vi "DaNISim.vi"(4 "Sonar offset angle":dbl, 5 "Action":enum16{"Init", "Run", "Release"}(ring), 6 "Sonar angle":dbl, 7 "Mode Select":T1(ring), 8 "error in (no error)":errorcluster, 9 "IP Adress":T2, 10 "Ul":dbl, 11 "Ur":dbl) -> (0 "error out":errorcluster, 1 "Sonar distance":dbl, 2 "OmegaL":dbl, 3 "OmegaR":dbl)   [LabVIEW 2016]
uses:
  <vilib>/userdefined/High Color/nirio_resource_hc.ctl
  <vilib>/robotics/Starter Kit/2.0/Sim Host Interface/NI_Robotics_Starter Kit Host_Sim_2.0.lvclass
  C:/Program Files (x86)/National Instruments/LabVIEW 2016/vi.lib/robotics/Starter Kit/Host Interface/NI_Robotics_Starter Kit Host.lvclass
  <vilib>/FPGAPlugInAG/sbRIO-9632/niLvFpga_Open_sbRIO-9632.vi
  <vilib>/rvi/interface/common/dynamic/niFpgaDynamicAddResources.vi
  <vilib>/Utility/error.llb/Error Cluster From Error Code.vi
  <vilib>/rvi/errors/niLvFpgaAdjustHostInterfaceError.vi
  <vilib>/FPGAPlugInAG/Dynamic/niLvFpga_Close_Dynamic.vi
  <vilib>/rvi/interface/nirviOpenFPGA/nirviOpenFPGA.xnode
  FPGA Bitfiles/StarterKit2.0Cus_FPGATarget_StarterKit2.0Cus_pLn805qeh78.lvbitx
  <vilib>/rvi/interface/nirviReadWriteControl/nirviReadWriteControl.xnode
  <vilib>/rvi/interface/nirviCloseFPGA/nirviCloseFPGA.xnode
  NiFpgaLv.dll
  <vilib>/rvi/interface/Simulation/niFpgaSimulationCallBeginRW.vi
  <vilib>/robotics/Simulator/NI_Robotics_Simulator.lvlib
  <vilib>/robotics/Starter Kit/Host Interface/NI_Robotics_Starter Kit Host.lvclass
panel:
  in  "N":i32=100
  in  "J":dbl=0.03
  in  "L":dbl=0.1825
  in  "R":dbl=0.046
  in  "M":dbl=3.0
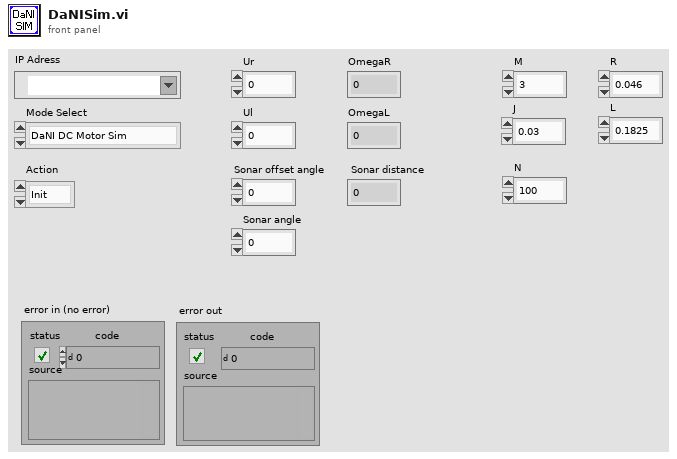
[diagram p1: front panel]
types:
  T1 = enum16{"DaNI DC Motor Sim", "DaNI Simulation", "DaNI Robot"}
  T2 = typedef "nirio_resource_hc.ctl" = tag
  T3 = cluster{"period (uSec)":u32, "pulse width (uSec)":u32}
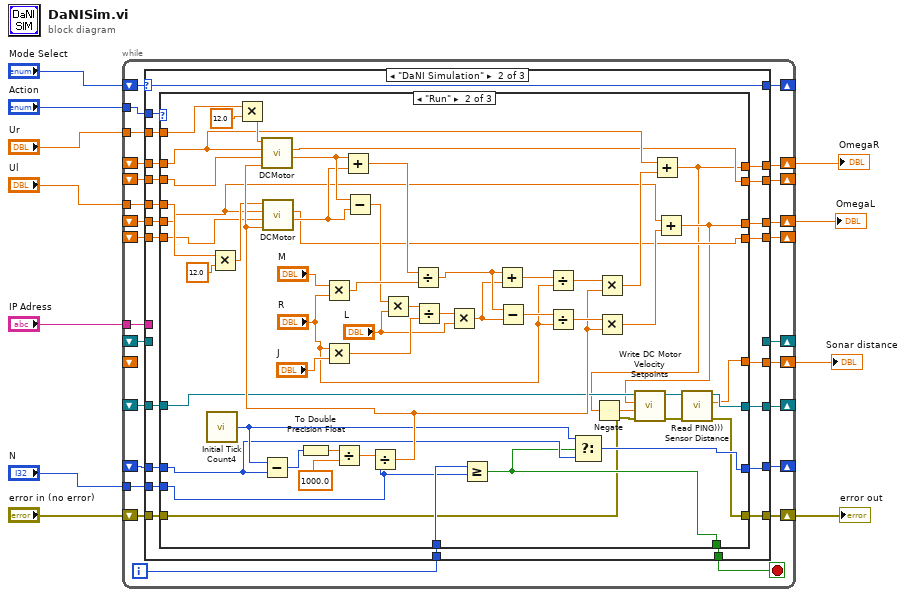
[diagram p0: block diagram]
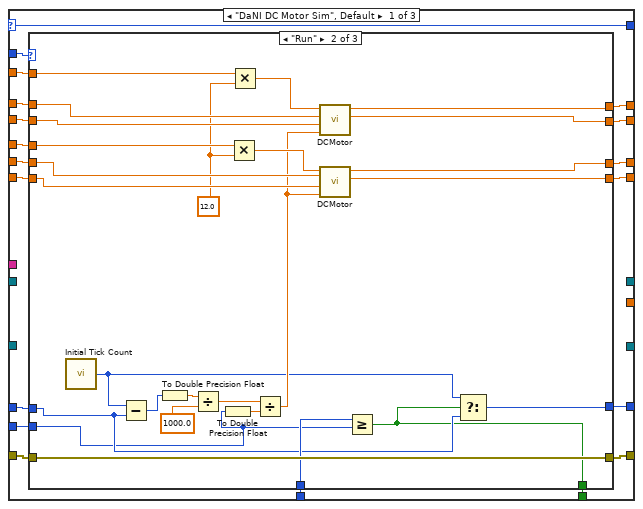
[diagram p2: hidden frame]
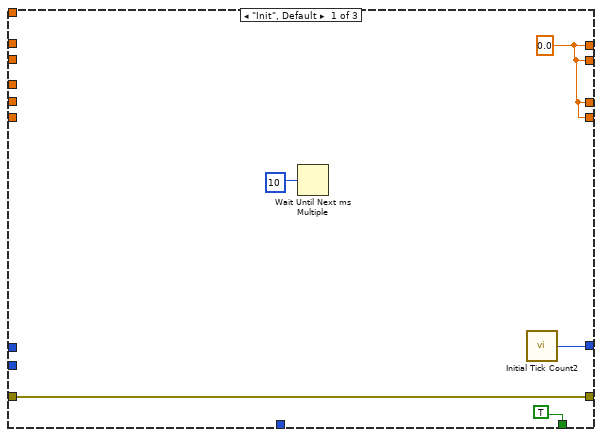
[diagram p3: hidden frame]
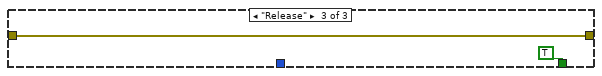
[diagram p4: hidden frame]
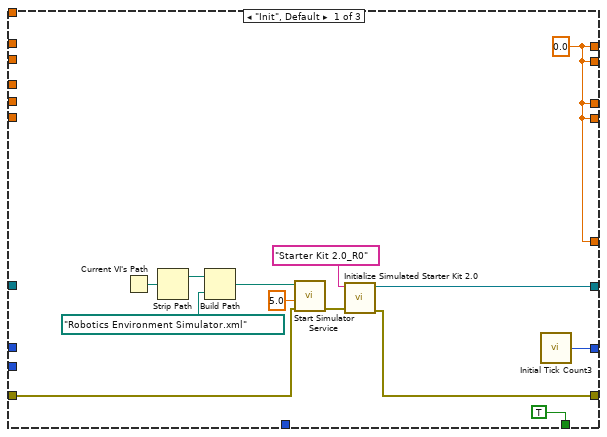
[diagram p5: hidden frame]
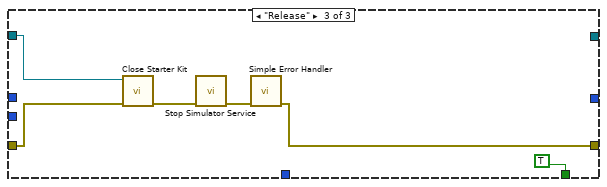
[diagram p6: hidden frame]
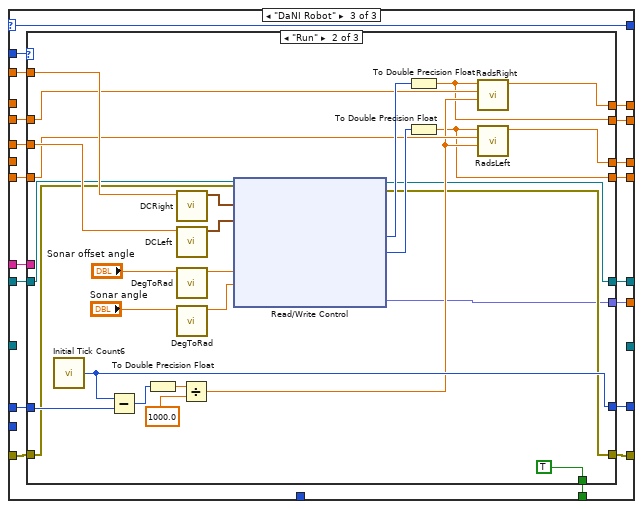
[diagram p7: hidden frame]
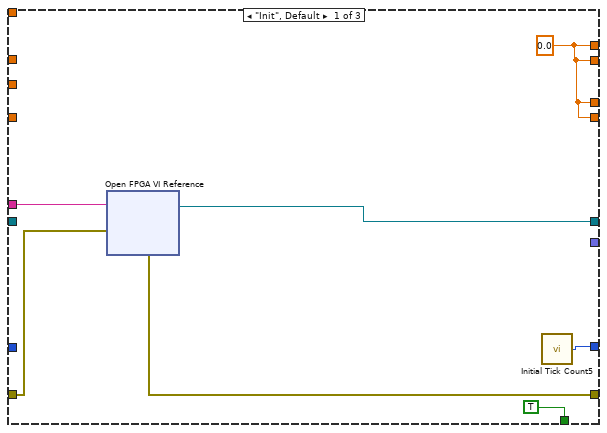
[diagram p8: hidden frame]
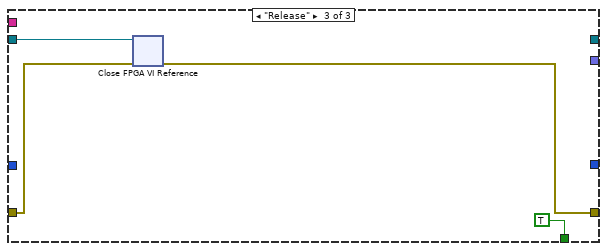
[diagram p9: hidden frame]
diagram:
  n1 = while {
    shift-right: [w35] -> w5
    shift-left: _ -> [w28]
    shift-right: [w34] -> _
    shift-left: _ -> [w27]
    tunnel: "Ur" -> [w29]
    shift-right: [w33] -> w4
    shift-left: _ -> [w25]
    shift-right: [w32] -> _
    shift-left: _ -> [w24]
    tunnel: "Ul" -> [w26]
    shift-right: [w30] -> _
    shift-left: _ -> [w31]
    shift-right: [w20] -> _
    shift-left: _ -> [w19]
    tunnel: "IP Adress" -> [w21]
    tunnel: "Action" -> [w36]
    shift-right: [w18] -> _
    shift-left: "Mode Select" -> [w37]
    tunnel: "N" -> [w17]
    shift-right: [w16] -> _
    shift-left: _ -> [w15]
    shift-right: [w14] -> w2
    shift-left: _ -> [_]
    shift-right: [w13] -> w1
    shift-left: "error in (no error)" -> [w12]
    i -> [w22]
    stop <- w23 stop-if-true
    n2 = case shown="\"DaNI Simulation\"" w37 {
      selector: w37 -> [w40 w94 w185]
      tunnel: w36 -> [w56 w107 w196]
      tunnel: [w55 w111 w202] -> w35
      tunnel: [w54 w110 w201] -> w34
      tunnel: [w53 w109 w200] -> w33
      tunnel: [w52 w108 w199] -> w32
      tunnel: w12 -> [w43 w105 w198]
      tunnel: [w42 w104 w197] -> w13
      tunnel: w31 -> [w51 w96 w188]
      tunnel: [w50 w103 w195] -> w30
      tunnel: w29 -> [w49 w102 w192]
      tunnel: w28 -> [w48 w101 _]
      tunnel: w27 -> [w47 w100 w190]
      tunnel: w26 -> [w46 w99 w191]
      tunnel: w25 -> [w45 w97 _]
      tunnel: w24 -> [w44 w98 w189]
      tunnel: [w41 w106 w186] -> w23
      tunnel: w22 -> [w39 w95 _]
      tunnel: w21 -> [_ _ w194]
      tunnel: [_ _ w193] -> w20
      tunnel: w19 -> [_ _ w187]
      tunnel: [w40 w94 w185] -> w18
      tunnel: w17 -> [w38 w93 _]
      tunnel: [_ w92 _] -> w16
      tunnel: w15 -> [_ w91 _]
      tunnel: [_ w90 w184] -> w14
      frame "DaNI DC Motor Sim", Default {
        n3 = case shown="\"Run\"" w56 {
          tunnel: [w61 w76 _] -> w55
          tunnel: [w61 w75 _] -> w54
          tunnel: [w61 w74 _] -> w53
          tunnel: [w61 w73 _] -> w52
          tunnel: w51 -> [_ w67 _]
          tunnel: [w58 w65 _] -> w50
          tunnel: w49 -> [_ w82 _]
          tunnel: w48 -> [_ w81 _]
          tunnel: w47 -> [_ w80 _]
          tunnel: w46 -> [_ w79 _]
          tunnel: w45 -> [_ w78 _]
          tunnel: w44 -> [_ w77 _]
          tunnel: w43 -> [w59 w72 w89]
          tunnel: [w59 w72 w89] -> w42
          tunnel: [TRUE w66 TRUE] -> w41
          tunnel: w39 -> [_ w69 _]
          tunnel: w38 -> [_ w64 _]
          frame "Init", Default {
            w61 = 0.0
            n4 = Wait Until Next ms Multiple(millisecond multiple=u32 10) -> ()  [unwired: 1 out]
            n5 = call "Initial Tick Count2"() -> ("Tick Count(mSec)"=w58:u32)
          }
          frame "Run" {
            w63 = 12.0 ("y")
            n6 = call "Initial Tick Count"() -> ("Tick Count(mSec)"=w68:u32)
            n7 = Subtract(x=w68, y=w67) -> (x-y=w87:u32)
            n8 = To Double Precision Float(number=w87) -> (double precision float=w85:dbl)
            n9 = Divide(x=w85, y=1000.0) -> (x/y=w71:dbl)
            n10 = To Double Precision Float(number=w64) -> (double precision float=w62:dbl)
            n11 = Multiply(x=w79, y=w63) -> (x*y=w83:dbl)
            n12 = Multiply(x=w82, y=w63) -> (x*y=w84:dbl)
            n13 = Divide(x=w71, y=w62) -> (x/y=w70:dbl)
            n14 = call "DCMotor.vi"("dt"=w70, "I"=w80, "Omega"=w81, "V"=w84) -> ("I Out"=w75:dbl, "Omega Out"=w76:dbl)  [unwired: 5 in, 1 out]
            n15 = call "DCMotor.vi"("dt"=w70, "I"=w77, "Omega"=w78, "V"=w83) -> ("I Out"=w73:dbl, "Omega Out"=w74:dbl)  [unwired: 5 in, 1 out]
            n16 = Greater Or Equal?(x=w69, y=w64) -> (x >= y?=w66:bool)
            n17 = Select(t=w68, s=w66, f=w67) -> (s? t:f=w65:u32)
          }
          frame "Release" {
          }
        }
      }
      frame "DaNI Simulation" {
        n18 = case shown="\"Run\"" w107 {
          tunnel: [w114 w132 _] -> w111
          tunnel: [w114 w141 _] -> w110
          tunnel: [w114 w133 _] -> w109
          tunnel: [w114 w140 _] -> w108
          tunnel: [TRUE w137 TRUE] -> w106
          tunnel: w105 -> [w113 w130 w180]
          tunnel: [w112 w126 w179] -> w104
          tunnel: [w123 w138 _] -> w103
          tunnel: w102 -> [_ w147 _]
          tunnel: w101 -> [_ w146 _]
          tunnel: w100 -> [_ w145 _]
          tunnel: w99 -> [_ w144 _]
          tunnel: w98 -> [_ w143 _]
          tunnel: w97 -> [_ w142 _]
          tunnel: w96 -> [_ w139 _]
          tunnel: w95 -> [_ w136 _]
          tunnel: w93 -> [_ w135 _]
          tunnel: [w115 w128 _] -> w92
          tunnel: w91 -> [_ w134 w178]
          tunnel: [w114 w127 _] -> w90
          frame "Init", Default {
            w114 = 0.0
            n19 = Current VI's Path() -> (path=w119:path)
            n20 = Strip Path(path=w119) -> (stripped path=w120:path)  [unwired: 1 out]
            n21 = Build Path(base path=w120, name or relative path=path "Robotics Environment Simulator.xml" ("manifest file")) -> (appended path=w122:path)
            n22 = call <vilib>:"Start Simulator Service.vi"("error in (no error)"=w113, "step size (ms)"=5.0, "manifest file"=w122) -> ("error out"=w117:errorcluster)  [unwired: 8 in]
            n23 = call <vilib>:"Initialize Simulated Starter Kit 2.0.vi"("error in (no error)"=w117, "robot ID"="Starter Kit 2.0_R0") -> ("error out"=w112:errorcluster, "simulated starter kit host 2.0 out"=w115:refnum<class "NI_Robotics_Starter Kit Host_Sim_2.0.lvclass">)  [unwired: 8 in]
            n24 = call "Initial Tick Count3"() -> ("Tick Count(mSec)"=w123:u32)
          }
          frame "Run" {
            n25 = call "Initial Tick Count4"() -> ("Tick Count(mSec)"=w152:u32)
            n26 = Multiply(x=w144, y=12.0) -> (x*y=w148:dbl)
            n27 = Multiply(x=w147, y=12.0) -> (x*y=w150:dbl)
            n28 = Subtract(x=w152, y=w139) -> (x-y=w175:u32)
            n29 = To Double Precision Float(number=w175) -> (double precision float=w177:dbl)
            n30 = Multiply(x="M", y="R") -> (x*y=w169:dbl)
            n31 = Multiply(x="R", y="J") -> (x*y=w166:dbl)
            n32 = Divide(x=w177, y=1000.0) -> (x/y=w154:dbl)
            n33 = Divide(x=w154, y=w135) -> (x/y=w153:dbl)
            n34 = call "DCMotor.vi"("dt"=w153, "I"=w145, "Omega"=w146, "V"=w150) -> ("Torque Out"=w172:dbl, "I Out"=w141:dbl)  [unwired: 5 in, 1 out]
            n35 = call "DCMotor.vi"("dt"=w153, "I"=w143, "Omega"=w142, "V"=w148) -> ("Torque Out"=w171:dbl, "I Out"=w140:dbl)  [unwired: 5 in, 1 out]
            n36 = Add(x=w172, y=w171) -> (x+y=w170:dbl)
            n37 = Subtract(x=w172, y=w171) -> (x-y=w168:dbl)
            n38 = Multiply(x=w168, y="L") -> (x*y=w167:dbl)
            n39 = Divide(x=w170, y=w169) -> (x/y=w163:dbl)
            n40 = Divide(x=w167, y=w166) -> (x/y=w165:dbl)
            n41 = Multiply(x=w165, y="L") -> (x*y=w162:dbl)
            n42 = Greater Or Equal?(x=w136, y=w135) -> (x >= y?=w137:bool)
            n43 = Add(x=w163, y=w162) -> (x+y=w161:dbl)
            n44 = Subtract(x=w163, y=w162) -> (x-y=w160:dbl)
            n45 = Divide(x=w161, y="R") -> (x/y=w158:dbl)
            n46 = Divide(x=w160, y="R") -> (x/y=w157:dbl)
            n47 = Select(t=w152, s=w137, f=w139) -> (s? t:f=w138:u32)
            n48 = Multiply(x=w158, y=w153) -> (x*y=w156:dbl)
            n49 = Multiply(x=w157, y=w153) -> (x*y=w155:dbl)
            n50 = Add(x=w146, y=w156) -> (x+y=w132:dbl)
            n51 = Negate(x=w132) -> (-x=w125:dbl)
            n52 = Add(x=w142, y=w155) -> (x+y=w133:dbl)
            n53 = call <vilib>:"Write DC Motor Velocity Setpoints.vi"("error in (no error)"=w130, "right motor ccw velocity (rad/s)"=w125, "left motor ccw velocity (rad/s)"=w133, "starter kit host in"=w134) -> ("error out"=w129:errorcluster, "starter kit host out"=w131:refnum<class "NI_Robotics_Starter Kit Host_Sim_2.0.lvclass">)  [unwired: 6 in]
            n54 = call <vilib>:"Read PING))) Sensor Distance.vi"("error in (no error)"=w129, "starter kit host in"=w131) -> ("error out"=w126:errorcluster, "distance (m)"=w127:dbl, "starter kit host out"=w128:refnum<class "NI_Robotics_Starter Kit Host_Sim_2.0.lvclass">)  [unwired: 6 in, 1 out]
          }
          frame "Release" {
            n55 = call-dynamic "Close Starter Kit.vi"("error in (no error)"=w180, "starter kit host in"=w178) -> ("error out"=w181:errorcluster)  [unwired: 9 in]
            n56 = call <vilib>:"Stop Simulator Service.vi"("error in (no error)"=w181) -> ("error out"=w182:errorcluster)  [unwired: 10 in]
            n57 = call <vilib>:"Simple Error Handler.vi"("error in (no error)"=w182) -> ("error out"=w179:errorcluster)  [unwired: 4 in, 4 out]
          }
        }
      }
      frame "DaNI Robot" {
        n58 = case shown="\"Run\"" w196 {
          tunnel: [w209 w233 _] -> w202
          tunnel: [w209 w211 _] -> w201
          tunnel: [w209 w231 _] -> w200
          tunnel: [w209 w210 _] -> w199
          tunnel: w198 -> [w205 w220 w239]
          tunnel: [w204 w219 w238] -> w197
          tunnel: [w208 w223 _] -> w195
          tunnel: w194 -> [w207 _ _]
          tunnel: [w206 w218 _] -> w193
          tunnel: w192 -> [_ w235 _]
          tunnel: w191 -> [_ w234 _]
          tunnel: w190 -> [_ w229 _]
          tunnel: w189 -> [_ w228 _]
          tunnel: w188 -> [_ w224 _]
          tunnel: w187 -> [_ w221 w240]
          tunnel: [TRUE TRUE TRUE] -> w186
          tunnel: [_ w212 _] -> w184
          frame "Init", Default {
            w209 = 0.0
            n59 = xnode "Open FPGA VI Reference"("error in"=w205, "resource name"=w207) -> ("FPGA VI Reference Out"=w206:refnum<k20>, "error out"=w204:errorcluster)
            n60 = call "Initial Tick Count5"() -> ("Tick Count(mSec)"=w208:u32)
          }
          frame "Run" {
            n61 = call "Initial Tick Count6"() -> ("Tick Count(mSec)"=w223:u32)
            n62 = Subtract(x=w223, y=w224) -> (x-y=w227:u32)
            n63 = To Double Precision Float(number=w227) -> (double precision float=w225:dbl)
            n64 = call "DCRight.vi"("Dc In"=w235) -> ("PWM Right Motor"=w237:T3)  [unwired: 10 in]
            n65 = call "DCLeft.vi"("Dc In"=w234) -> ("PWM Left Motor"=w236:T3)  [unwired: 10 in]
            n66 = call "DegToRad.vi"("Degrees"="Sonar offset angle") -> ("Radians"=w216:dbl)  [unwired: 10 in]
            n67 = call "DegToRad.vi"("Degrees"="Sonar angle") -> ("Radians"=w213:dbl)  [unwired: 10 in]
            n68 = Divide(x=w225, y=1000.0) -> (x/y=w222:dbl)
            n69 = xnode "Read/Write Control"("FPGA VI Reference In"=w221, "error in"=w220, "PWM Right Motor"=w237, "PWM Left Motor"=w236, "hs400_0_ccw offset"=w216, "hs400_0_ccw angle"=w213) -> ("FPGA VI Reference Out"=w218:refnum<k20>, "error out"=w219:errorcluster, "Right cw count (pulses)"=w232:i32, "Left cw count (pulses)"=w230:i32, "PING)))_0_dist"=w212:fxp<+,32,8>)
            n70 = To Double Precision Float(number=w232) -> (double precision float=w211:dbl)
            n71 = To Double Precision Float(number=w230) -> (double precision float=w210:dbl)
            n72 = call "RadsRight.vi"("dt"=w222, "Cw2"=w229, "Cw1"=w211) -> ("Rs"=w233:dbl)  [unwired: 8 in]
            n73 = call "RadsLeft.vi"("dt"=w222, "Cw2"=w228, "Cw1"=w210) -> ("Rs"=w231:dbl)  [unwired: 8 in]
          }
          frame "Release" {
            n74 = xnode "Close FPGA VI Reference"("FPGA VI Reference In"=w240, "error in"=w239) -> ("error out"=w238:errorcluster)
          }
        }
      }
    }
  }
  "OmegaR" <- w5
  "error out" <- w1
  "OmegaL" <- w4
  "Sonar distance" <- w2
